vi "GetTagByDataGroup.vi"(8 "error in (no error)":errorcluster, 10 "data group":string, 11 "matches":T1[](array[typedef])) -> (0 "error out":errorcluster, 3 "Tag":T1)   [LabVIEW 2017]
uses:
  <vilib>/addons/InsightCM/MessageBus/Base/controls/Tag.ctl
  <vilib>/addons/InsightCM/MessageBus/Base/controls/KeyValuePair.ctl
  <vilib>/addons/InsightCM/Utilities/PropertyHelpers/PropertyHelpers.lvlib
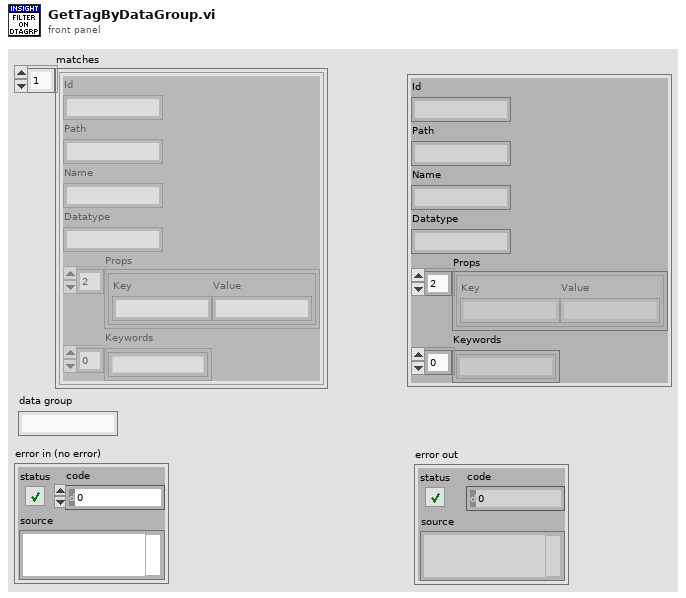
[diagram p1: front panel]
types:
  T1 = typedef "Tag.ctl" = cluster{"Id":string, "Path":string, "Name":string, "Datatype":string, "Props":T2[], "Keywords":string[]}
  T2 = typedef "KeyValuePair.ctl" = cluster{"Key":string, "Value":string}
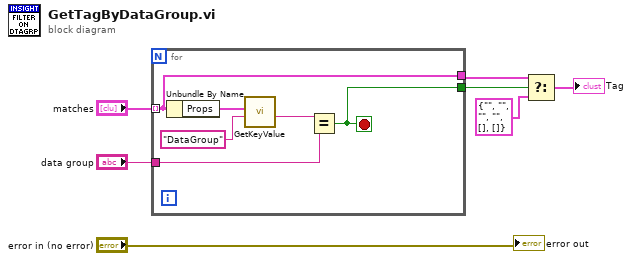
[diagram p0: block diagram]
diagram:
  n1 = for {
    tunnel: "matches" -> [w9] mode=indexing
    tunnel: "data group" -> [w10]
    tunnel: [w9] -> w2
    tunnel: [w8] -> w4
    stop <- w8 stop-if-true
    n2 = Unbundle By Name(w9) -> ("Props"=w13:T2[])
    n3 = call <vilib>:"GetKeyValue.vi"("key"="DataGroup", "key value pairs"=w13) -> ("value"=w11:string)  [unwired: 7 in, 2 out]
    n4 = Equal?(x=w11, y=w10) -> (x = y?=w8:bool)
  }
  n5 = Select(t=w2, s=w4, f=T1 {"Id"="", "Path"="", "Name"="", "Datatype"="", "Props"=[], "Keywords"=[]} ("Tag")) -> (s? t:f=→"Tag":T1)
  "error out" <- "error in (no error)"
